vi "Get Self.vi"(11 "Addresses Strategy in":refnum<class "Addresses Strategy.lvclass">) -> (2 "Self":refnum<user-event>)   [LabVIEW 2021, in "jettl.lvlib" / "Addresses Strategy.lvlib" / "Addresses Strategy.lvclass"]
uses:
  Addresses Strategy.lvclass
  Msg/Msg.lvclass
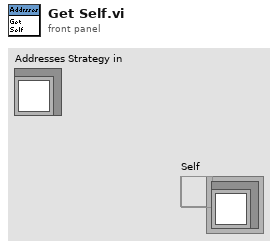
[diagram p1: front panel]
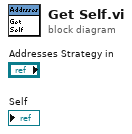
[diagram p0: block diagram]
diagram:
